vi "CreatePublicEvents.vi"(8 "error in (no error)":errorcluster, 11 "Measurement.WavelengthSweeping":refnum<class "Measurement.WavelengthSweeping.lvclass">) -> (0 "error out":errorcluster, 3 "Measurement.WavelengthSweeping out":refnum<class "Measurement.WavelengthSweeping.lvclass">)   [LabVIEW 2017, in "Measurement.WavelengthSweeping.lvclass"]
doc: "---------------------------------------------------------------\nJKI State Machine Objects™\nhttp://jki.net/state-machine-objects/\nCopyright (C) 2005-2015, JKI <info@jki.net>\nALL RIGHTS RESERVEDJKI State Machine Objects (SMO) 1.0.0.5\nJKI - JKI\nCopyright (c) 2016, JKI"
uses:
  Measurement.WavelengthSweeping.lvclass
  Typedefs/DataChanged--EventData--Cluster.ctl
  Measurement.WavelengthSweeping.lvclass/Measurement.WavelengthSweeping.ctl
  <vilib>/JKI/JKI SMO/SMO/SMO.lvclass
panel:
  # "For instructions on how to use the JKI State Machine Objects, examples and video tutorials, visit:\nhttp://jki.net/state-machine-objects/\n\nJKI State Machine Objects™\nhttp://jki.net/state-machine-objects/\nCopyright (C) 2005-2015, JKI <info@jki.net>\nALL RIGHTS RESERVED"
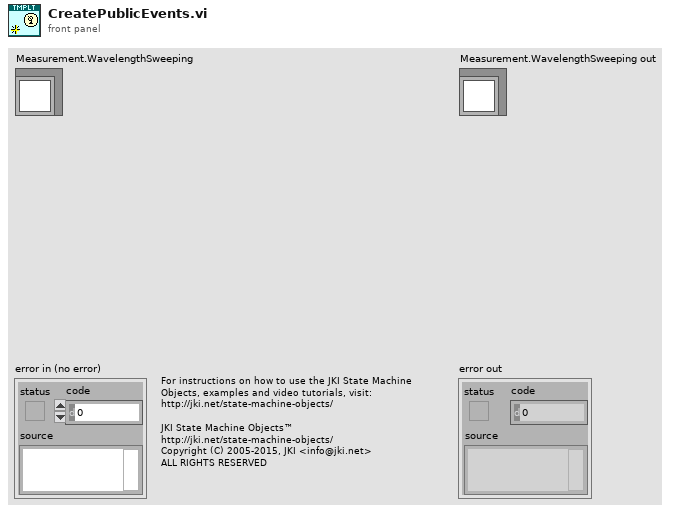
[diagram p1: front panel]
types:
  T1 = typedef "Measurement.WavelengthSweeping.lvclass/DataChanged--EventData--Cluster.ctl" = cluster{"Timestamp":timestamp, "Old Value":string, "New Value":string}
  T2 = typedef "Measurement.WavelengthSweeping.lvclass/PrivateData--Ref.ctl" = refnum<data-value>
  T3 = typedef "Measurement.WavelengthSweeping.lvclass/PrivateData--Cluster.ctl" = cluster{"Configuration":T4, "Public Events":T5, "Protected Events":T6, "Data":string}
  T4 = typedef "Measurement.WavelengthSweeping.lvclass/Configuration--Cluster.ctl" = cluster{"Suffix":string}
  T5 = typedef "Measurement.WavelengthSweeping.lvclass/PublicEvents--Cluster.ctl" = cluster{"Data Changed":refnum<user-event>}
  T6 = typedef "Measurement.WavelengthSweeping.lvclass/ProtectedEvents--Cluster.ctl" = cluster{"API_Template":refnum<user-event>}
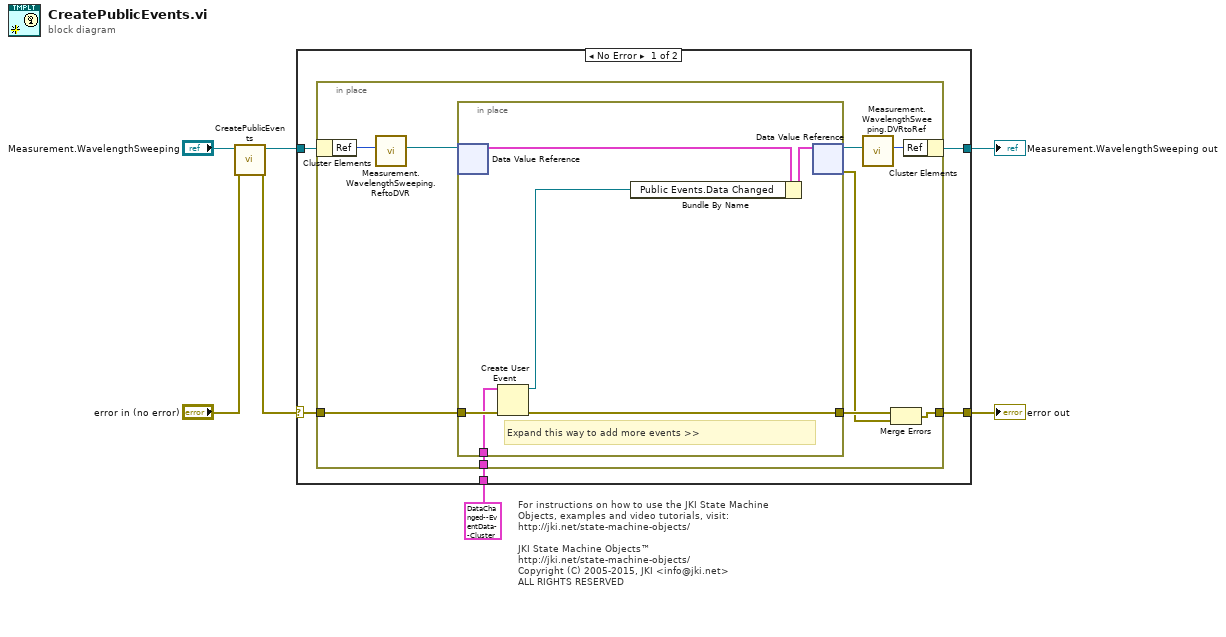
[diagram p0: block diagram]
diagram:
  # "For instructions on how to use the JKI State Machine Objects, examples and video tutorials, visit:\nhttp://jki.net/state-machine-objects/\n\nJKI State Machine Objects™\nhttp://jki.net/state-machine-objects/\nCopyright (C) 2005-2015, JKI <info@jki.net>\nALL RIGHTS RESERVED"
  n1 = call-parent "CreatePublicEvents.vi"("error in (no error)"="error in (no error)", "SMO"="Measurement.WavelengthSweeping") -> ("error out"=w1:errorcluster, "SMO out"=w3:refnum<class "Measurement.WavelengthSweeping.lvclass">)  [unwired: 8 in]
  n2 = case shown="No Error" w1 {
    selector: w1 -> [w10 w29]
    tunnel: [w9 w29] -> w6
    tunnel: [w11 w28] -> w7
    tunnel: w3 -> [w12 w28]
    tunnel: T1 {"Timestamp"=timestamp(0 s since 1904-01-01), "Old Value"="", "New Value"=""} ("Data In Event Data") -> [w8 _]
    frame No Error {
      n3 = in-place {
        in-place-border: w10 -> [w21]
        in-place-border: [w18] -> w9
        in-place-border: w8 -> [w17]
        n4 = in-place-cluster #1(w12) -> ("Ref"=w16:u32)
        n5 = call "Measurement.WavelengthSweeping.ReftoDVR.vi"("Ref"=w16) -> ("Ref"=w15:T2)  [unwired: 10 in]
        n6 = in-place {
          in-place-border: w21 -> [w24]
          in-place-border: [w25] -> w20
          in-place-border: w17 -> [w23]
          # "Expand this way to add more events >>"
          n7 = in-place-dvr #2(w15) -> (w26:T3)  [unwired: 1 out]
          n8 = Create User Event(user event datatype=w23, error in=w24) -> (user event=w22:refnum<user-event>, error out=w25:errorcluster)
          n9 = Bundle By Name(cluster=w26, "Public Events.Data Changed"=w22) -> (w27:T3)
          n10 = in-place-dvr #2(w27) -> (w14:T2, w19:errorcluster)
        }
        n11 = call "Measurement.WavelengthSweeping.DVRtoRef.vi"("Ref"=w14) -> ("Ref"=w13:u32)  [unwired: 10 in]
        n12 = Merge Errors(w20, w19) -> (w18:errorcluster)
        n13 = in-place-cluster #1("Ref"=w13) -> (w11:refnum<class "Measurement.WavelengthSweeping.lvclass">)
      }
    }
    frame Error {
    }
  }
  "error out" <- w6
  "Measurement.WavelengthSweeping out" <- w7
